vi "Attitude Control Close.vi"(8 "error in (no error)":errorcluster, 11 "Attitude Control Handle":T1) -> (0 "error out":errorcluster)   [LabVIEW 2015, in "RDS Libraries.lvlib" / "lv-attitudecontrol.lvlib"]
uses:
  lv-attitudecontrol.lvlib
  Controls/AttitudeHandle.ctl
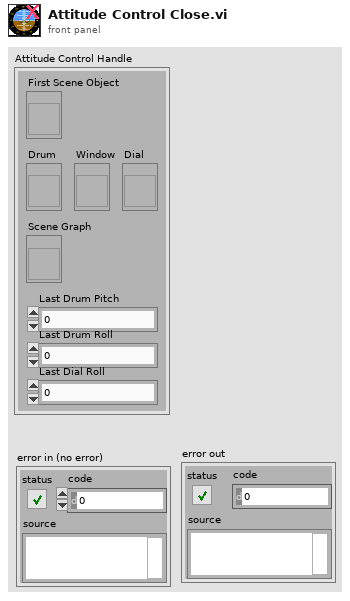
[diagram p1: front panel]
types:
  T1 = typedef "RDS Libraries.lvlib/lv-attitudecontrol.lvlib/AttitudeHandle.ctl" = cluster{"First Scene Object":refnum<vi>, "Drum":refnum<vi>, "Window":refnum<vi>, "Dial":refnum<vi>, "Scene Graph":refnum<vi>, "Last Drum Pitch":dbl, "Last Drum Roll ":dbl, "Last Dial Roll":dbl}
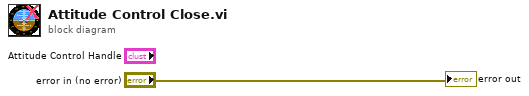
[diagram p0: block diagram]
diagram:
  "error out" <- "error in (no error)"
